vi "User Message Teststand Event Callback.vi"(4 "GUI.lvlib:Auto UI.lvlib:Auto UI.lvclass":refnum<class "Auto UI.lvclass">, 5 "Event Data":cluster{"uiMsg":refnum<k7>}, 6 "Control Ref":refnum<k7>, 7 "Event Common Data":T1) -> ()   [LabVIEW 2023, in "GUI.lvlib" / "Auto UI.lvlib" / "Auto UI.lvclass"]
uses:
  Auto UI.lvclass
  Typdefs/Auto GUI/Software Description.ctl
  Auto UI.lvclass/Auto UI.ctl
  GUI.lvlib
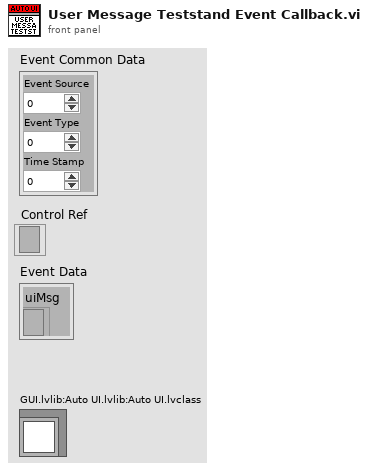
[diagram p1: front panel]
types:
  T1 = cluster{"Event Source":i32, "Event Type":u32, "Time Stamp":u32}
  T2 = typedef "GUI.lvlib/Software Description.ctl" = cluster{"Test SW Version:":string, "VAL SW Version:":string}
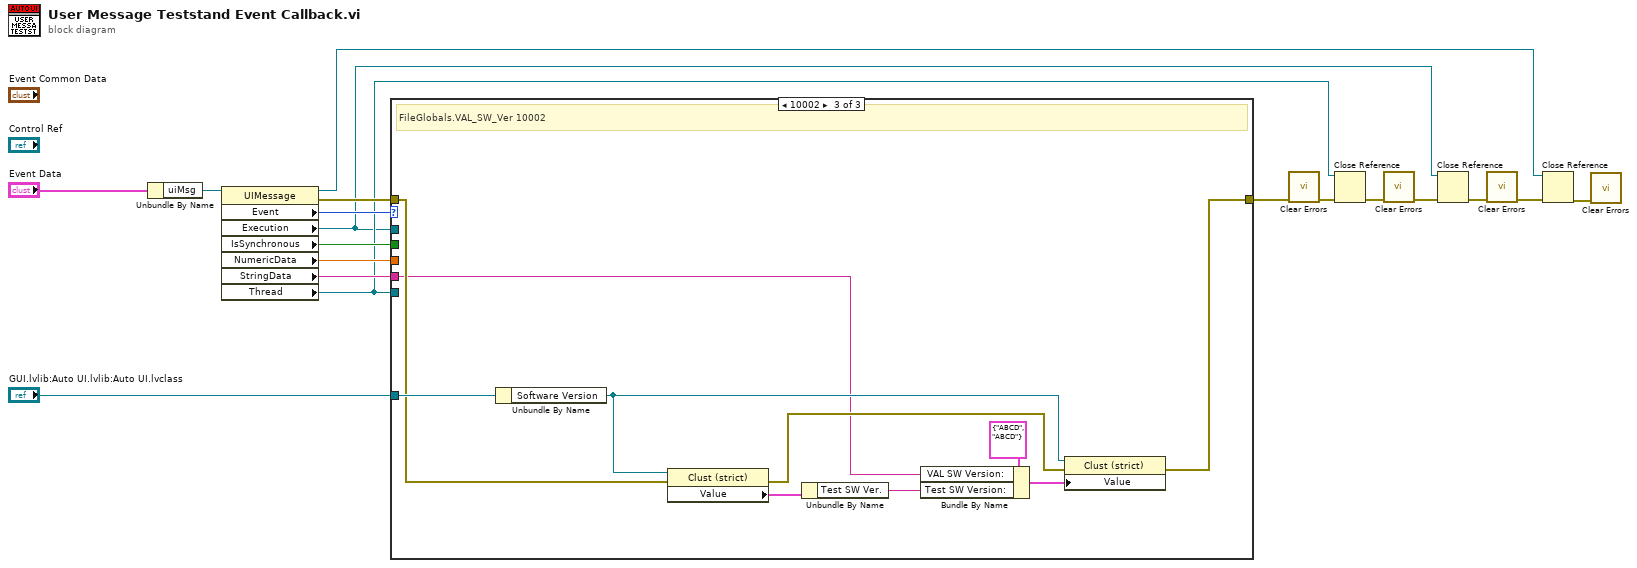
[diagram p0: block diagram]
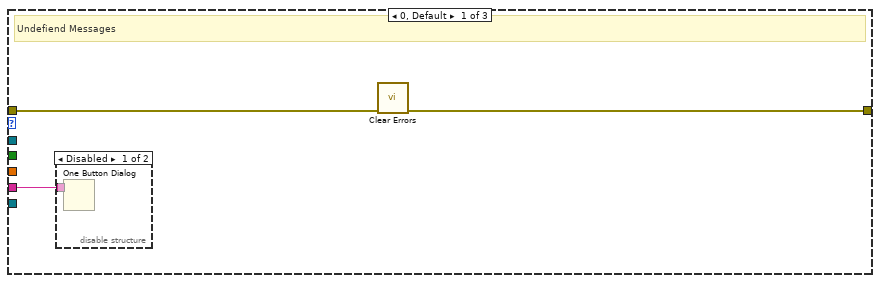
[diagram p2: hidden frame]
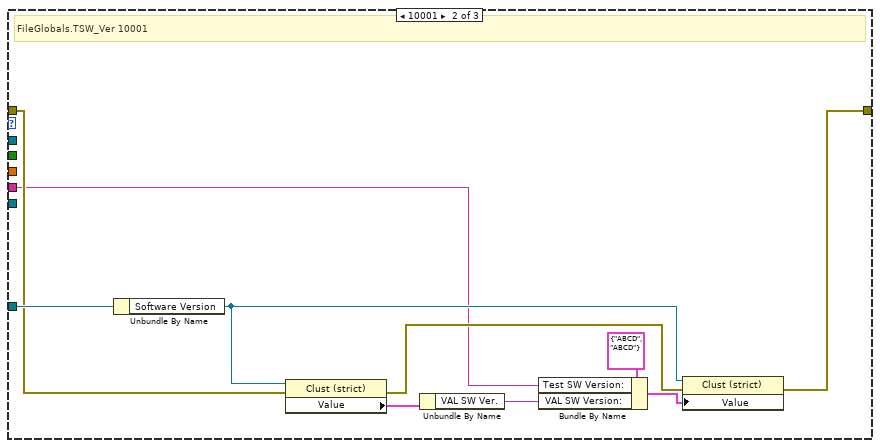
[diagram p4: hidden frame]
diagram:
  n1 = Unbundle By Name("Event Data") -> ("uiMsg"=w18:refnum<k7>)
  n2 = property class="UIMessage"(reference=w18) -> (reference out=w13:refnum<k7>, error out=w11:errorcluster, "Event"=w17:i32, "Execution"=w3:refnum<k7>, "IsSynchronous"=w16:bool, "NumericData"=w15:dbl, "StringData"=w14:string, "Thread"=w4:refnum<k7>)  [unwired: 1 in]
  n3 = case shown="10002" w17 {
    tunnel: w3 -> [_ _ _]
    tunnel: w16 -> [_ _ _]
    tunnel: w15 -> [_ _ _]
    tunnel: w14 -> [w19 w23 w33]
    tunnel: w4 -> [_ _ _]
    tunnel: "GUI.lvlib:Auto UI.lvlib:Auto UI.lvclass" -> [_ w32 w42]
    tunnel: [w20 w25 w35] -> w5
    tunnel: w11 -> [w21 w28 w38]
    frame 0, Default {
      # "Undefiend Messages"
      n4 = disable-structure shown="Disabled" {
        disable-tunnel: w19 -> [w22 _]
        frame Disabled {
          n5 = One Button Dialog(message=w22) -> ()  [unwired: 1 in, 1 out]
        }
        frame Enabled {
        }
      }
      n6 = call <vilib>:"Clear Errors.vi"("error in (no error)"=w21) -> ("error out"=w20:errorcluster)  [unwired: 5 in, 1 out]
    }
    frame 10001 {
      # "FileGlobals.TSW_Ver 10001"
      n7 = Unbundle By Name(w32) -> ("Software Version"=w24:refnum<vi>)
      n8 = property class="Clust (strict)"(reference=w24, error in=w28) -> (error out=w27:errorcluster, "Value"=w30:T2)  [unwired: 1 out]
      n9 = Unbundle By Name(w30) -> ("VAL SW Ver."=w29:string)
      n10 = Bundle By Name(cluster=T2 {"Test SW Version:"="ABCD", "VAL SW Version:"="ABCD"} ("Value"), "Test SW Version:"=w23, "VAL SW Version:"=w29) -> (w26:T2)
      n11 = property class="Clust (strict)"(reference=w24, error in=w27, "Value"=w26) -> (error out=w25:errorcluster)  [unwired: 1 out]
    }
    frame 10002 {
      # "FileGlobals.VAL_SW_Ver 10002"
      n12 = Unbundle By Name(w42) -> ("Software Version"=w34:refnum<vi>)
      n13 = property class="Clust (strict)"(reference=w34, error in=w38) -> (error out=w37:errorcluster, "Value"=w40:T2)  [unwired: 1 out]
      n14 = Unbundle By Name(w40) -> ("Test SW Ver."=w39:string)
      n15 = Bundle By Name(cluster=T2 {"Test SW Version:"="ABCD", "VAL SW Version:"="ABCD"} ("Value"), "VAL SW Version:"=w33, "Test SW Version:"=w39) -> (w36:T2)
      n16 = property class="Clust (strict)"(reference=w34, error in=w37, "Value"=w36) -> (error out=w35:errorcluster)  [unwired: 1 out]
    }
  }
  n17 = call <vilib>:"Clear Errors.vi"("error in (no error)"=w5) -> ("error out"=w8:errorcluster)  [unwired: 5 in, 1 out]
  n18 = Close Reference(reference=w4, error in (no error)=w8) -> (error out=w7:errorcluster)
  n19 = call <vilib>:"Clear Errors.vi"("error in (no error)"=w7) -> ("error out"=w9:errorcluster)  [unwired: 5 in, 1 out]
  n20 = Close Reference(reference=w3, error in (no error)=w9) -> (error out=w10:errorcluster)
  n21 = call <vilib>:"Clear Errors.vi"("error in (no error)"=w10) -> ("error out"=w6:errorcluster)  [unwired: 5 in, 1 out]
  n22 = Close Reference(reference=w13, error in (no error)=w6) -> (error out=w12:errorcluster)
  n23 = call <vilib>:"Clear Errors.vi"("error in (no error)"=w12) -> ()  [unwired: 5 in, 2 out]
